vi "字符串控件字号自适应.vi"(6 "留白（7）":i16=7, 7 "新旧尺寸信息":T1, 8 "错误输入（无错误）":errorcluster, 11 "字符串控件-引用":refnum<vi>) -> (0 "错误输出":errorcluster, 3 "字号":u32)   [LabVIEW 2017, in "项目开发助手.lvlib" / "UI助手.lvlib"]
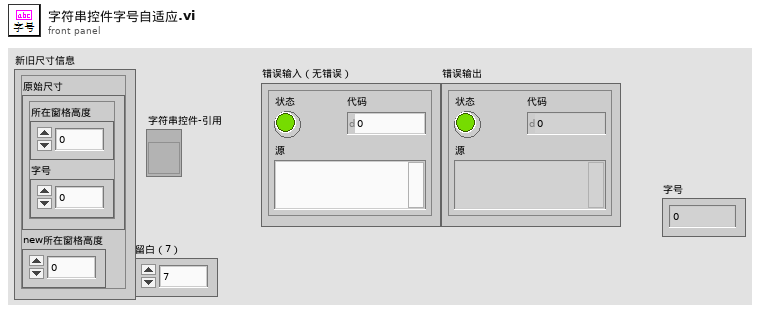
[diagram p1: front panel]
types:
  T1 = cluster{"原始尺寸":cluster{"所在窗格高度":u32, "字号":u32}, "new所在窗格高度":u32}
  T2 = typedef "LVRectTypeDef.ctl" = cluster{"Left":i16, "Top":i16, "Right":i16, "Bottom":i16}
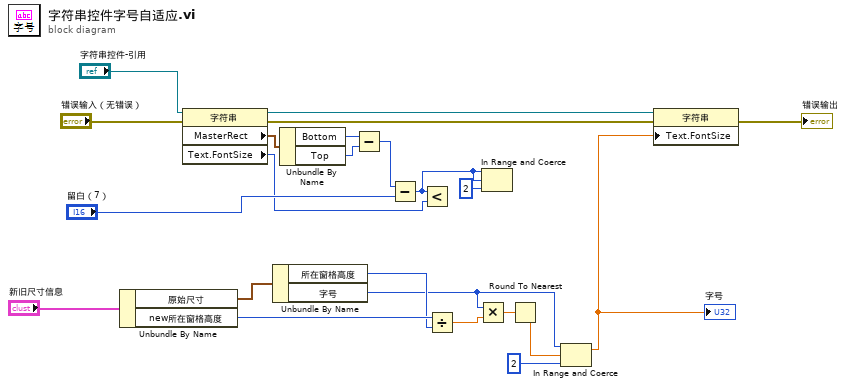
[diagram p0: block diagram]
diagram:
  n1 = Unbundle By Name("新旧尺寸信息") -> ("原始尺寸"=w9:cluster{"所在窗格高度":u32, "字号":u32}, "new所在窗格高度"=w8:u32)
  n2 = property class="字符串"(reference="字符串控件-引用", error in="错误输入（无错误）") -> (reference out=w22:refnum<vi>, error out=w23:errorcluster, "MasterRect"=w21:T2, "Text.FontSize"=w13:u32)
  n3 = Unbundle By Name(w9) -> ("所在窗格高度"=w7:u32, "字号"=w2:u32)
  n4 = Unbundle By Name(w21) -> ("Bottom"=w18:i16, "Top"=w17:i16)
  n5 = Subtract(x=w18, y=w17) -> (x-y=w19:i16)
  n6 = Subtract(x=w19, y="留白（7）") -> (x-y=w11:i16)
  n7 = Less?(x=w11, y=w13) -> ()  [unwired: 1 out]
  n8 = Divide(x=w8, y=w7) -> (x/y=w6:dbl)
  n9 = Multiply(x=w2, y=w6) -> (x*y=w5:dbl)
  n10 = In Range and Coerce(upper limit=w11, x=w11, lower limit=i16 2 ("下限")) -> ()  [unwired: 2 out]
  n11 = Round To Nearest(number=w5) -> (nearest integer value=w3:dbl)
  n12 = In Range and Coerce(upper limit=w2, x=w3, lower limit=i16 2 ("下限")) -> (coerced(x)=w1:dbl)  [unwired: 1 out]
  "字号" <- w1
  n13 = property class="字符串"(reference=w22, error in=w23, "Text.FontSize"=w1) -> (error out=→"错误输出":errorcluster)  [unwired: 1 out]
